vi "BuildWriteFrame.vi"(11 "String in":string) -> (3 "String out":string)   [LabVIEW 2023]
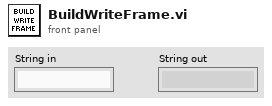
[diagram p1: front panel]
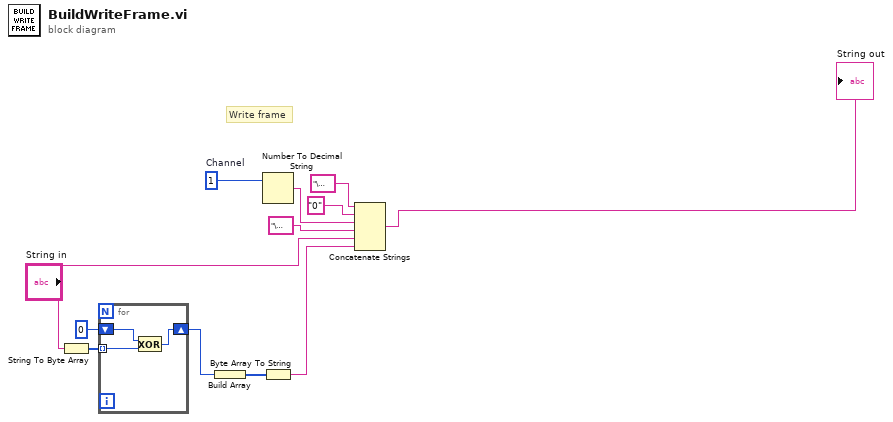
[diagram p0: block diagram]
diagram:
  w2 = 1  # Channel
  # "Write frame"
  n1 = String To Byte Array(string="String in") -> (unsigned byte array=w6:u8[])
  n2 = for {
    tunnel: w6 -> [w14] mode=indexing
    shift-right: [w13] -> w8
    shift-left: 0 -> [w15]
    n3 = Exclusive Or(1:w14, 2:w15) -> (0:w13:i32)
  }
  n4 = Build Array(w8) -> (w9:i32[])
  n5 = Number To Decimal String(number=w2) -> (decimal integer string=w3:string)  [unwired: 1 in]
  n6 = Byte Array To String(unsigned byte array=w9) -> (string=w12:string)
  n7 = Concatenate Strings("\u0004" ("string"), "0" ("string"), w3, "\u0002" ("string"), "String in", w12) -> (→"String out":string)
